vi "CLSUIP_GetApplicationOfClass.vi"(8 "error in (no error)":errorcluster, 11 "LVClassLibrary Ref":refnum<vi>) -> (0 "error out":errorcluster, 2 "Application":refnum<vi>, 3 "LVClassLibrary Ref out":refnum<vi>)   [LabVIEW 2021]
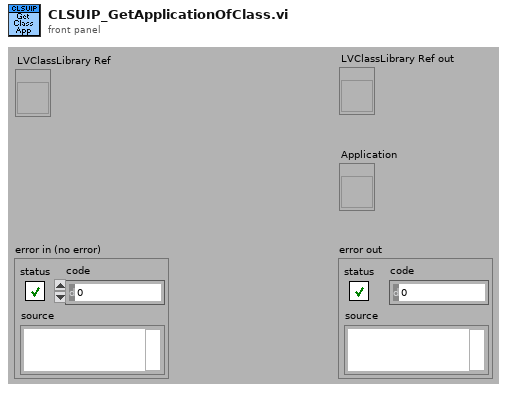
[diagram p1: front panel]
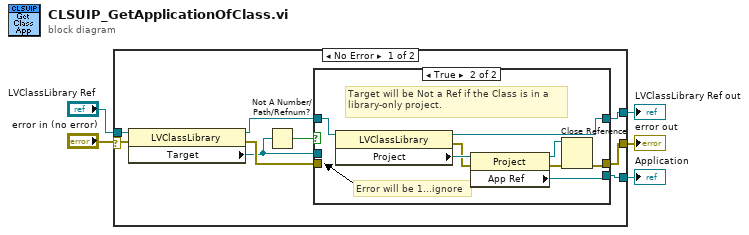
[diagram p0: block diagram]
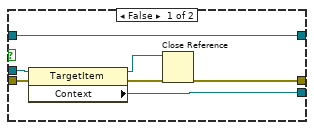
[diagram p2: hidden frame]
diagram:
  n1 = case shown="No Error" "error in (no error)" {
    selector: "error in (no error)" -> [w6 w30]
    tunnel: [w14 _] -> w5
    tunnel: [w13 w30] -> w4
    tunnel: "LVClassLibrary Ref" -> [w11 w31]
    tunnel: [w7 w31] -> w2
    frame No Error {
      n2 = property class="LVClassLibrary"(reference=w11, error in=w6) -> (reference out=w8:refnum<vi>, error out=w12:errorcluster, "Target"=w10:refnum<vi>)
      n3 = Not A Number/Path/Refnum?(number/path/refnum=w10) -> (NaN/Path/Refnum?=w9:bool)
      n4 = case shown="True" w9 {
        tunnel: [w21 w26] -> w14
        tunnel: [w16 w23] -> w13
        tunnel: w12 -> [w19 _]
        tunnel: w10 -> [w18 _]
        tunnel: w8 -> [w17 w29]
        tunnel: [w17 w24] -> w7
        frame False {
          n5 = property class="TargetItem"(reference=w18, error in=w19) -> (reference out=w15:refnum<vi>, error out=w20:errorcluster, "Context"=w21:refnum<vi>)
          n6 = Close Reference(reference=w15, error in (no error)=w20) -> (error out=w16:errorcluster)
        }
        frame True {
          # "Error will be 1...ignore"
          # "Target will be Not a Ref if the Class is in a \nlibrary-only project."
          n7 = property class="LVClassLibrary"(reference=w29) -> (reference out=w24:refnum<vi>, error out=w27:errorcluster, "Project"=w28:refnum<vi>)  [unwired: 1 in]
          n8 = property class="Project"(reference=w28, error in=w27) -> (reference out=w22:refnum<vi>, error out=w25:errorcluster, "App Ref"=w26:refnum<vi>)
          n9 = Close Reference(reference=w22, error in (no error)=w25) -> (error out=w23:errorcluster)
        }
      }
    }
    frame Error {
    }
  }
  "Application" <- w5
  "error out" <- w4
  "LVClassLibrary Ref out" <- w2
